vi "Set Slit Width.vi"(8 "error in (no error)":errorcluster, 10 "Slit Width (um)":dbl, 11 "SpectraPro in":refnum<class "SpectraPro.lvclass">) -> (0 "error out":errorcluster, 2 "Slit Width (um) out":dbl, 3 "SpectraPro out":refnum<class "SpectraPro.lvclass">)   [LabVIEW 2019, in "SpectraPro.lvclass"]
uses:
  SpectraPro.lvclass
  SpectraPro.lvclass/SpectraPro.ctl
  SpectraPro-LabVIEW-Driver/SpectraPro.lvlib
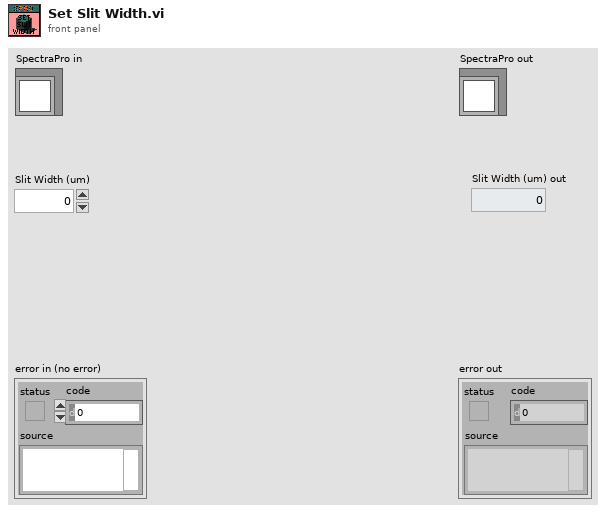
[diagram p1: front panel]
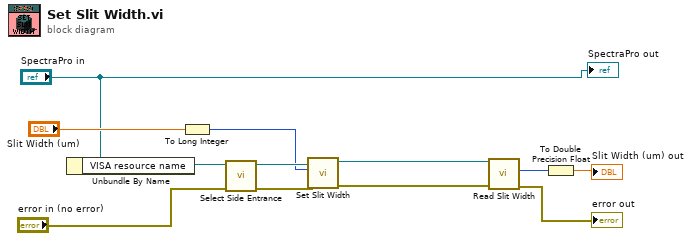
[diagram p0: block diagram]
diagram:
  n1 = Unbundle By Name("SpectraPro in") -> ("VISA resource name"=w5:refnum<visa-resource-name>)
  n2 = To Long Integer(number="Slit Width (um)") -> (32bit integer=w3:i32)
  n3 = call "Select Side Entrance.vi"("error in (no error)"="error in (no error)", "VISA resource name"=w5) -> ("error out"=w7:errorcluster, "VISA resource name out"=w6:refnum<visa-resource-name>)  [unwired: 7 in, 1 out]
  n4 = call "Set Slit Width.vi"("error in (no error)"=w7, "Slit Width (um)"=w3, "VISA resource name"=w6) -> ("error out"=w2:errorcluster, "VISA resource name out"=w1:refnum<visa-resource-name>)  [unwired: 6 in, 1 out]
  n5 = call "Read Slit Width.vi"("error in (no error)"=w2, "VISA resource name"=w1) -> ("error out"=→"error out":errorcluster, "Slit Width (um)"=w10:i32)  [unwired: 6 in, 2 out]
  n6 = To Double Precision Float(number=w10) -> (double precision float=→"Slit Width (um) out":dbl)
  "SpectraPro out" <- "SpectraPro in"
